vi "Build DashBoard Data.vi"(11 "Dashboard Enables":T3={"Analog Module 1"=[TRUE, TRUE, TRUE, TRUE, TRUE, TRUE, TRUE, TRUE], "Analog Module 2"=[FALSE, FALSE, FALSE, FALSE, FALSE, FALSE, FALSE, FALSE], "Digital Module 1"=TRUE, "Digital Module 2"=FALSE, "Solenoid Module"=TRUE}) -> ()   [LabVIEW 2011]
doc: "This VI builds data and sends it back to the dashboard PC program. By default it sends back the raw values for the first analog, digital, and solenoid module. Modify it to send back the data you want to view. Consider adding higher level data to the Dashboard Datatype.ctl and to this VI. Then update the Dashboard to display the data however you like.\n\nThis software is licensed. Open the labview\\readme\\WPI Robotics Library Open Source License.txt file for more information."
uses:
  DashboardEnable.ctl
  Dashboard Datatype.ctl
  <vilib>/Rock Robotics/WPI/DriverStation/WPI_DriverStationDigitalData.ctl
panel:
  out "Dashboard Data":T1
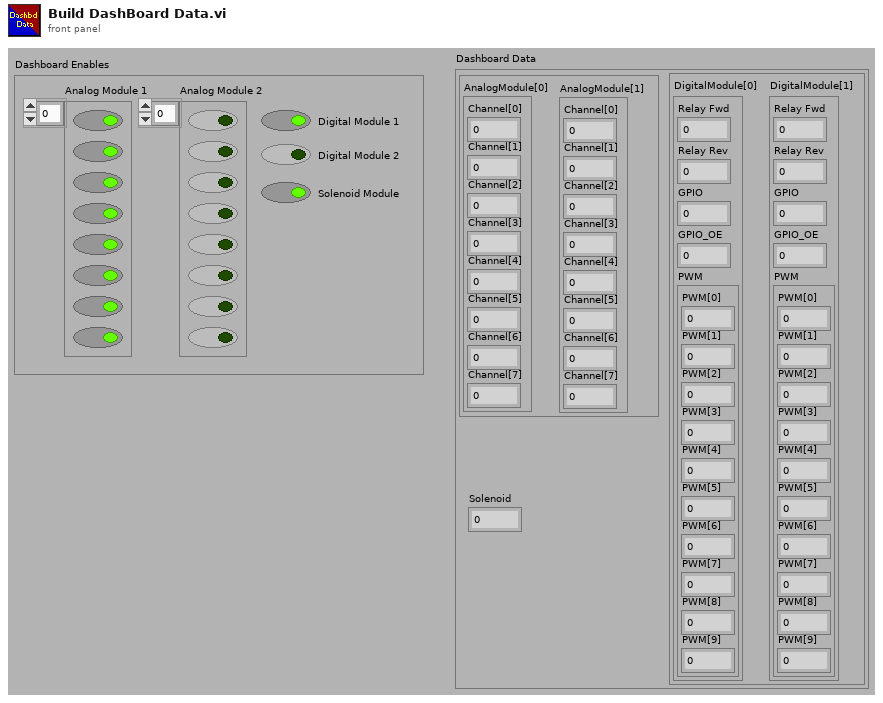
[diagram p1: front panel]
types:
  T1 = typedef "Dashboard Datatype.ctl" = cluster{cluster{"AnalogModule[0]":cluster{"Channel[0]":sgl, "Channel[1]":sgl, "Channel[2]":sgl, "Channel[3]":sgl, "Channel[4]":sgl, "Channel[5]":sgl, "Channel[6]":sgl, "Channel[7]":sgl}, "AnalogModule[1]":cluster{"Channel[0]":sgl, "Channel[1]":sgl, "Channel[2]":sgl, "Channel[3]":sgl, "Channel[4]":sgl, "Channel[5]":sgl, "Channel[6]":sgl, "Channel[7]":sgl}}, cluster{"DigitalModule[0]":T2, "DigitalModule[1]":T2}, "Solenoid":u8}
  T2 = typedef "WPI_DriverStationDigitalData.ctl" = cluster{"Relay Fwd":u8, "Relay Rev":u8, "GPIO":u16, "GPIO_OE":u16, "PWM":cluster{"PWM[0]":u8, "PWM[1]":u8, "PWM[2]":u8, "PWM[3]":u8, "PWM[4]":u8, "PWM[5]":u8, "PWM[6]":u8, "PWM[7]":u8, "PWM[8]":u8, "PWM[9]":u8}}
  T3 = typedef "DashboardEnable.ctl" = cluster{"Analog Module 1":bool[], "Analog Module 2":bool[], "Digital Module 1":bool, "Digital Module 2":bool, "Solenoid Module":bool}
  T4 = cluster{"AnalogModule[0]":cluster{"Channel[0]":sgl, "Channel[1]":sgl, "Channel[2]":sgl, "Channel[3]":sgl, "Channel[4]":sgl, "Channel[5]":sgl, "Channel[6]":sgl, "Channel[7]":sgl}, "AnalogModule[1]":cluster{"Channel[0]":sgl, "Channel[1]":sgl, "Channel[2]":sgl, "Channel[3]":sgl, "Channel[4]":sgl, "Channel[5]":sgl, "Channel[6]":sgl, "Channel[7]":sgl}}
  T5 = cluster{"Channel[0]":sgl, "Channel[1]":sgl, "Channel[2]":sgl, "Channel[3]":sgl, "Channel[4]":sgl, "Channel[5]":sgl, "Channel[6]":sgl, "Channel[7]":sgl}[]
  T6 = cluster{"Channel[0]":sgl, "Channel[1]":sgl, "Channel[2]":sgl, "Channel[3]":sgl, "Channel[4]":sgl, "Channel[5]":sgl, "Channel[6]":sgl, "Channel[7]":sgl}
  T7 = cluster{"AnalogModule[0][0]":sgl, "AnalogModule[0][1]":sgl, "AnalogModule[0][2]":sgl, "AnalogModule[0][3]":sgl, "AnalogModule[0][4]":sgl, "AnalogModule[0][5]":sgl, "AnalogModule[0][6]":sgl, "AnalogModule[0][7]":sgl}
  T8 = cluster{"[0]":cluster{"Channel[0]":sgl, "Channel[1]":sgl, "Channel[2]":sgl, "Channel[3]":sgl, "Channel[4]":sgl, "Channel[5]":sgl, "Channel[6]":sgl, "Channel[7]":sgl}, "[1]":cluster{"Channel[0]":sgl, "Channel[1]":sgl, "Channel[2]":sgl, "Channel[3]":sgl, "Channel[4]":sgl, "Channel[5]":sgl, "Channel[6]":sgl, "Channel[7]":sgl}}
  T9 = cluster{"DigitalModule[0]":T2, "DigitalModule[1]":T2}
  T10 = typedef "FPGA_DIODevRef.ctl" = cluster{"DevStatus":errorcluster, "Module":T11}
  T11 = typedef "FPGA_TypedefDigitalModule.ctl" = enum16{"Digital Module 1", "Digital Module 2"}
  T12 = cluster{"[0]":u8, "[1]":u8, "[2]":u8, "[3]":u8, "[4]":u8, "[5]":u8, "[6]":u8, "[7]":u8, "[8]":u8, "[9]":u8}
  T13 = typedef "FPGA_SolenoidDevRef.ctl" = cluster{"DevStatus":errorcluster, "Module":T14}
  T14 = typedef "FPGA_TypedefSolenoidModule.ctl" = enum16{"Solenoid Module 1", "Solenoid Module 2"}
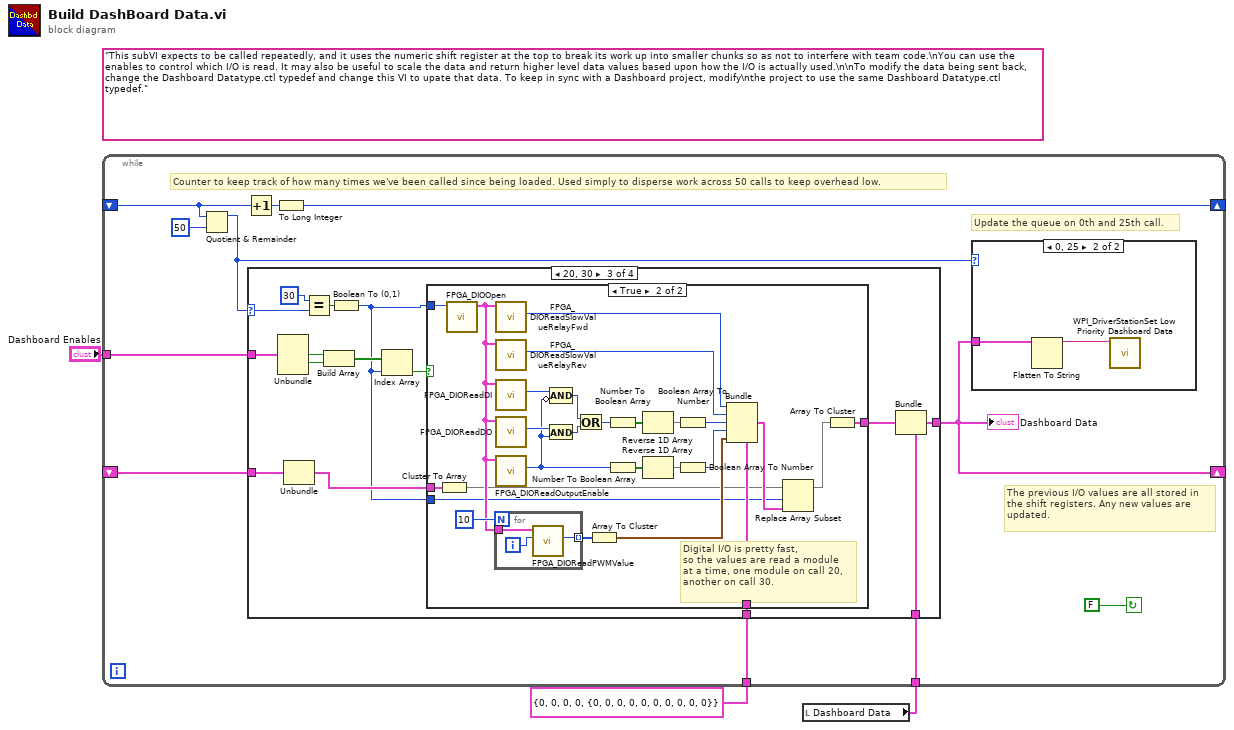
[diagram p0: block diagram]
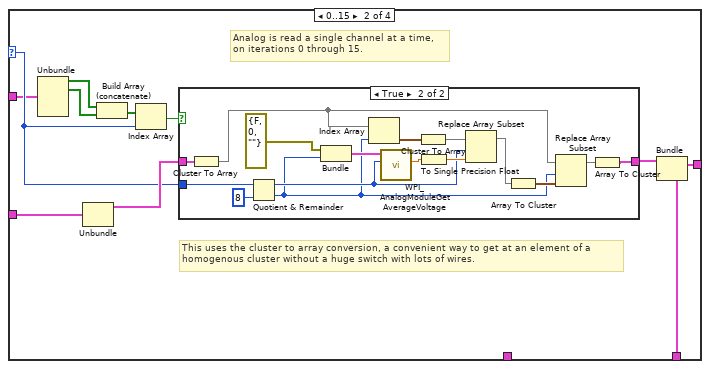
[diagram p4: hidden frame]
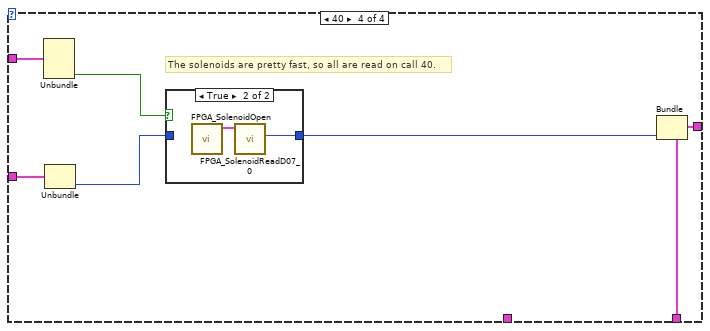
[diagram p7: hidden frame]
diagram:
  (unwired) "This subVI expects to be called repeatedly, and it uses the numeric shift register at the top to break its work up into smaller chunks so as not to interfere with team code.\nYou can use the enables to control which I/O is read. It may also be useful to scale the data and return higher level data values based upon how the I/O is actually used.\n\nTo modify the data being sent back, change the Dashboard Datatype.ctl typedef and change this VI to upate that data. To keep in sync with a Dashboard project, modify\nthe project to use the same Dashboard Datatype.ctl typedef."
  n1 = local read "Dashboard Data"() -> (w2:T1)
  n2 = while {
    shift-right: [w7] -> _
    shift-left: _ -> [w9]
    shift-right: [w4] -> _
    shift-left: _ -> [w12]
    tunnel: T2 {"Relay Fwd"=0, "Relay Rev"=0, "GPIO"=0, "GPIO_OE"=0, "PWM"={"PWM[0]"=0, "PWM[1]"=0, "PWM[2]"=0, "PWM[3]"=0, "PWM[4]"=0, "PWM[5]"=0, "PWM[6]"=0, "PWM[7]"=0, "PWM[8]"=0, "PWM[9]"=0}} ("DigitalModule[1]") -> [w11]
    tunnel: w2 -> [w6]
    tunnel: "Dashboard Enables" -> [w5]
    stop <- FALSE continue-if-true
    # "Counter to keep track of how many times we've been called since being loaded. Used simply to disperse work across 50 calls to keep overhead low."
    # "Update the queue on 0th and 25th call."
    # "The previous I/O values are all stored in\nthe shift registers. Any new values are\nupdated."
    n3 = Quotient & Remainder(x=w9, y=50) -> (x-y*floor(x/y)=w8:i32)  [unwired: 1 out]
    n4 = Increment(x=w9) -> (x+1=w14:i32)
    n5 = case shown="20, 30" w8 {
      selector: w8 -> [_ w23 w56 _]
      tunnel: [w17 w19 w47 w94] -> w4
      tunnel: w12 -> [w17 w18 w49 w96]
      tunnel: w11 -> [_ _ w60 _]
      tunnel: w6 -> [_ w25 w48 w93]
      tunnel: w5 -> [_ w22 w54 w97]
      frame Default {
        # "Don't update any I/O"
      }
      frame 0..15 {
        # "This uses the cluster to array conversion, a convenient way to get at an element of a\nhomogenous cluster without a huge switch with lots of wires."
        # "Analog is read a single channel at a time,\non iterations 0 through 15."
        n6 = Unbundle(w22) -> ("Analog Module 1"=w21:bool[], "Analog Module 2"=w20:bool[])  [unwired: 3 out]
        n7 = Unbundle(w18) -> (w24:T4)  [unwired: 2 out]
        n8 = Build Array (concatenate)(w21, w20) -> (w27:bool[])
        n9 = Index Array(array=w27, index=w23) -> (element=w28:bool)
        n10 = case shown="True" w28 {
          tunnel: w23 -> [_ w36]
          tunnel: [w29 w33] -> w26
          tunnel: w24 -> [w29 w32]
          frame False {
          }
          frame True {
            n11 = Cluster To Array(cluster=w32) -> (array=w31:T5)
            n12 = Quotient & Remainder(x=w36, y=8) -> (x-y*floor(x/y)=w35:i32, floor(x/y)=w30:i32)
            n13 = Bundle("DevStatus"=errorcluster {"status"=FALSE, "code"=0, "source"=""}, w30) -> (w44:cluster{"DevStatus":errorcluster, i32})  [unwired: 1 out]
            n14 = Index Array(array=w31, index=w30) -> (element=w38:T6)
            n15 = call <vilib>:"WPI_AnalogModuleGetAverageVoltage.vi"("Channel"=w35, "AnalogModuleDevStatus"=w44) -> ("Average Voltage"=w41:dbl)  [unwired: 1 in, 8 out]
            n16 = Cluster To Array(cluster=w38) -> (array=w37:sgl[])
            n17 = To Single Precision Float(number=w41) -> (single precision float=w40:sgl)
            n18 = Replace Array Subset(array=w37, new element=w40, index=w35) -> (w39:sgl[])
            n19 = Array To Cluster(array=w39) -> (cluster=w43:T7)
            n20 = Replace Array Subset(array=w31, new element=w43, index=w30) -> (w34:T5)
            n21 = Array To Cluster(array=w34) -> (cluster=w33:T8)
          }
        }
        n22 = Bundle(cluster=w25, w26) -> (w19:T1)  [unwired: 2 out]
      }
      frame 20, 30 {
        n23 = Unbundle(w54) -> ("Digital Module 1"=w53:bool, "Digital Module 2"=w52:bool)  [unwired: 3 out]
        n24 = Unbundle(w49) -> (w51:T9)  [unwired: 2 out]
        n25 = Equal?(x=30, y=w56) -> (x = y?=w58:bool)
        n26 = Build Array(w53, w52) -> (w55:bool[])
        n27 = Boolean To (0,1)(Boolean=w58) -> (0, 1=w46:i16)
        n28 = Index Array(array=w55, index=w46) -> (element=w57:bool)
        n29 = case shown="True" w57 {
          tunnel: w60 -> [_ w69]
          tunnel: [w61 w62] -> w50
          tunnel: w46 -> [_ w67]
          tunnel: w46 -> [_ w66]
          tunnel: w51 -> [w61 w65]
          frame False {
          }
          frame True {
            # "Digital I/O is pretty fast,\nso the values are read a module\nat a time, one module on call 20,\nanother on call 30."
            n30 = Cluster To Array(cluster=w65) -> (array=w64:T2[])
            n31 = call <vilib>:"FPGA_DIOOpen.vi"("Module (Module 1)"=w67) -> ("DIODeviceRef"=w85:T10)  [unwired: 1 in, 9 out]
            n32 = for {
              N: 10 -> [_]
              tunnel: w85 -> [w90]
              tunnel: [w88] -> w86 mode=indexing
              i -> [w89]
              n33 = call <vilib>:"FPGA_DIOReadPWMValue.vi"("PWMChannel"=w89, "DIODeviceRef In"=w90) -> ("PWMValue"=w88:u8)  [unwired: 1 in, 8 out]
            }
            n34 = call <vilib>:"FPGA_DIOReadSlowValueRelayFwd.vi"("DIODeviceRef In"=w85) -> ("Relay Forward"=w78:u8)  [unwired: 1 in, 9 out]
            n35 = call <vilib>:"FPGA_DIOReadSlowValueRelayRev.vi"("DIODeviceRef In"=w85) -> ("Relay Reverse"=w79:u8)  [unwired: 1 in, 9 out]
            n36 = call <vilib>:"FPGA_DIOReadDI.vi"("DIODeviceRef In"=w85) -> ("DI"=w83:u16)  [unwired: 1 in, 9 out]
            n37 = call <vilib>:"FPGA_DIOReadDO.vi"("DIODeviceRef In"=w85) -> ("DO"=w82:u16)  [unwired: 1 in, 9 out]
            n38 = call <vilib>:"FPGA_DIOReadOutputEnable.vi"("DIODeviceRef In"=w85) -> ("OutputEnable"=w73:u16)  [unwired: 1 in, 9 out]
            n39 = And(x=w82, y=w73) -> (x .and. y?=w81:u16)
            n40 = Compound Arithmetic op=AND(w83, invert w73) -> (w80:u16)
            n41 = Or(x=w80, y=w81) -> (x .or. y?=w71:u16)
            n42 = Array To Cluster(array=w86) -> (cluster=w84:T12)
            n43 = Number To Boolean Array(number=w71) -> (Boolean array=w76:bool[])
            n44 = Number To Boolean Array(number=w73) -> (Boolean array=w75:bool[])
            n45 = Reverse 1D Array(array=w76) -> (reversed array=w77:bool[])
            n46 = Reverse 1D Array(array=w75) -> (reversed array=w74:bool[])
            n47 = Boolean Array To Number(Boolean array=w77) -> (number=w70:u32)
            n48 = Boolean Array To Number(Boolean array=w74) -> (number=w72:u32)
            n49 = Bundle(cluster=w69, "Relay Fwd"=w78, "Relay Rev"=w79, "GPIO"=w70, "GPIO_OE"=w72, "PWM"=w84) -> (w68:T2)
            n50 = Replace Array Subset(array=w64, new element=w68, index=w66) -> (w63:T2[])
            n51 = Array To Cluster(array=w63) -> (cluster=w62:cluster{"[0]":T2, "[1]":T2})
          }
        }
        n52 = Bundle(cluster=w48, w50) -> (w47:T1)  [unwired: 2 out]
      }
      frame 40 {
        # "The solenoids are pretty fast, so all are read on call 40."
        n53 = Unbundle(w97) -> ("Solenoid Module"=w91:bool)  [unwired: 4 out]
        n54 = Unbundle(w96) -> ("Solenoid"=w95:u8)  [unwired: 2 out]
        n55 = case shown="True" w91 {
          tunnel: [w98 w99] -> w92
          tunnel: w95 -> [w98 _]
          frame False {
          }
          frame True {
            n56 = call <vilib>:"FPGA_SolenoidOpen.vi"() -> ("SolenoidDevRef"=w100:T13)  [unwired: 2 in, 9 out]
            n57 = call <vilib>:"FPGA_SolenoidReadD07_0.vi"("SolenoidDevRef"=w100) -> ("DO7:0"=w99:u8)  [unwired: 1 in, 9 out]
          }
        }
        n58 = Bundle(cluster=w93, "Solenoid"=w92) -> (w94:T1)  [unwired: 2 out]
      }
    }
    "Dashboard Data" <- w4
    n59 = To Long Integer(number=w14) -> (32bit integer=w7:i32)
    n60 = case shown="0, 25" w8 {
      tunnel: w4 -> [_ w16]
      frame Default {
      }
      frame 0, 25 {
        n61 = Flatten To String(anything=w16) -> (data string=w15:string)  [unwired: 1 in, 4 out]
        n62 = call <vilib>:"WPI_DriverStationSet Low Priority Dashboard Data.vi"("User Data"=w15) -> ()  [unwired: 1 in, 10 out]
      }
    }
  }
